vi "Update SubPanel.vi"(8 "error in (no error)":errorcluster, 9 "VI Refnum":refnum<vi>, 10 "Window Name":string, 11 "User Interface in":refnum<class "User Interface.lvclass">) -> (0 "error out":errorcluster, 3 "User Interface out":refnum<class "User Interface.lvclass">)   [LabVIEW 2017, in "User Interface.lvlib" / "User Interface.lvclass"]
uses:
  User Interface.lvclass
  User Interface.lvclass/User Interface.ctl
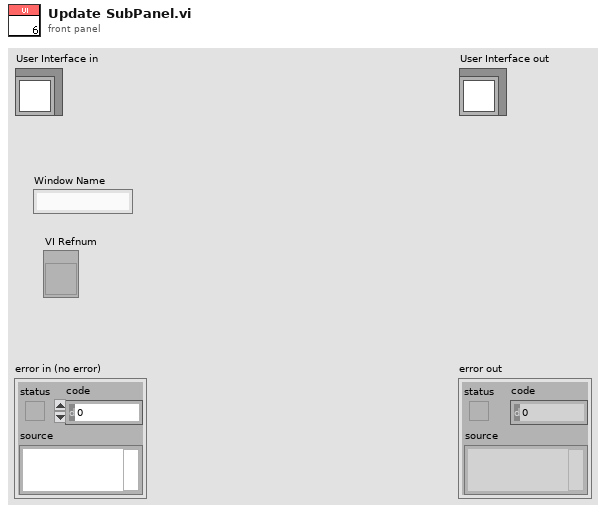
[diagram p1: front panel]
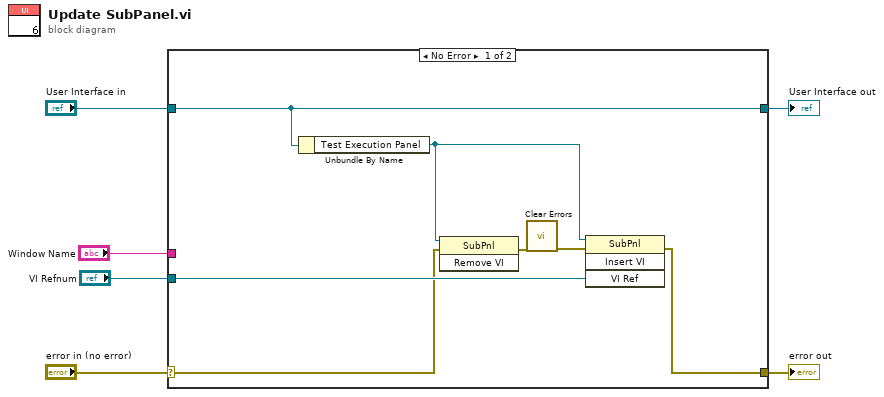
[diagram p0: block diagram]
diagram:
  n1 = case shown="No Error" "error in (no error)" {
    selector: "error in (no error)" -> [w8 w15]
    tunnel: [w7 w15] -> w5
    tunnel: [w13 w14] -> w3
    tunnel: "User Interface in" -> [w13 w14]
    tunnel: "Window Name" -> [_ _]
    tunnel: "VI Refnum" -> [w11 _]
    frame No Error {
      n2 = Unbundle By Name(w13) -> ("Test Execution Panel"=w10:refnum<vi>)
      n3 = invoke class="SubPnl" method="Remove VI"(reference=w10, error in=w8) -> (error out=w12:errorcluster)  [unwired: 1 in, 2 out]
      n4 = call <vilib>:"Clear Errors.vi"("error in (no error)"=w12) -> ("error out"=w9:errorcluster)  [unwired: 5 in, 1 out]
      n5 = invoke class="SubPnl" method="Insert VI"(reference=w10, error in=w9, "VI Ref"=w11) -> (error out=w7:errorcluster)  [unwired: 1 in, 3 out]
    }
    frame Error {
    }
  }
  "error out" <- w5
  "User Interface out" <- w3
